vi "GetConditionalReference.vi"(6 "error in":errorcluster, 9 "LoopTunnel in":refnum<class "LoopTunnel.lvclass">) -> (0 "error out":errorcluster, 3 "LoopTunnel out":refnum<class "LoopTunnel.lvclass">, 4 "UID":i32)   [LabVIEW 2014, in "LoopTunnel.lvclass"]
uses:
  LoopTunnel.lvclass
  LoopTunnel.lvclass/LoopTunnel.ctl
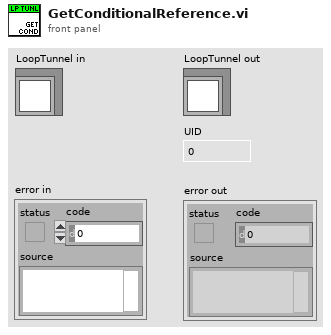
[diagram p1: front panel]
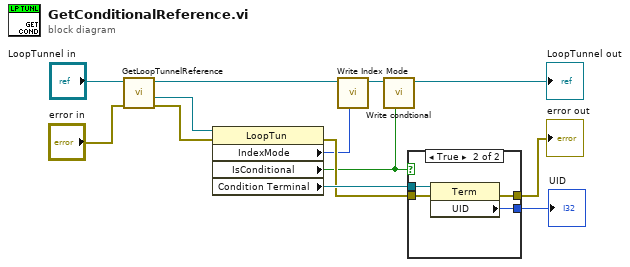
[diagram p0: block diagram]
diagram:
  n1 = call "GetLoopTunnelReference.vi"("error in"="error in", "LoopTunnel in"="LoopTunnel in") -> ("error out"=w11:errorcluster, "reference out"=w12:refnum<vi>, "LoopTunnel out"=w2:refnum<class "LoopTunnel.lvclass">)  [unwired: 7 in]
  n2 = property class="LoopTun"(reference=w12, error in=w11) -> (error out=w9:errorcluster, "IndexMode"=w4:u32, "IsConditional"=w1:bool, "Condition Terminal"=w10:refnum<vi>)  [unwired: 1 out]
  n3 = call "Write Index Mode.vi"("Index Mode"=w4, "LoopTunnel in"=w2) -> ("LoopTunnel out"=w5:refnum<class "LoopTunnel.lvclass">)  [unwired: 7 in]
  n4 = call "Write condtional.vi"("condtional"=w1, "LoopTunnel in"=w5) -> ("LoopTunnel out"=→"LoopTunnel out":refnum<class "LoopTunnel.lvclass">)  [unwired: 7 in]
  n5 = case shown="True" w1 {
    tunnel: w10 -> [_ w18]
    tunnel: w9 -> [w14 w17]
    tunnel: [w14 w16] -> w7
    tunnel: [_ w15] -> w6
    frame False {
    }
    frame True {
      n6 = property class="Term"(reference=w18, error in=w17) -> (error out=w16:errorcluster, "UID"=w15:i32)  [unwired: 1 out]
    }
  }
  "error out" <- w7
  "UID" <- w6
